vi "Prova selezionata.vi"() -> ()   [LabVIEW 2019]
panel:
  out "Prova selezionata":i16
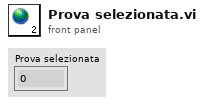
[diagram p1: front panel]
diagram:
